vi "Fuel Injector Stage Voltage Threshold.vi"(8 "error in (no error)":errorcluster, 11 "Node Ptr":T1 format="%.0x") -> (0 "error out":errorcluster)   [LabVIEW 2019, in "Fuel Injector Analysis Addon System Explorer.lvlib"]
uses:
  Fuel Injector Analysis Addon System Explorer.lvlib
  <vilib>/NI VeriStand/Custom Device API/Custom Device Item Ref.ctl
  <vilib>/NI VeriStand/Custom Device API/Custom Device API.lvlib
panel:
  out "Units":string
  in  "Default Value":dbl
  in  "SHDocVw.IWebBrowser":refnum<k7>(container)
  in  "Header":cluster{"Section Name":string}={"Section Name"="Custom Device Item Settings"}
  in  "Description":string
  out "Name":string
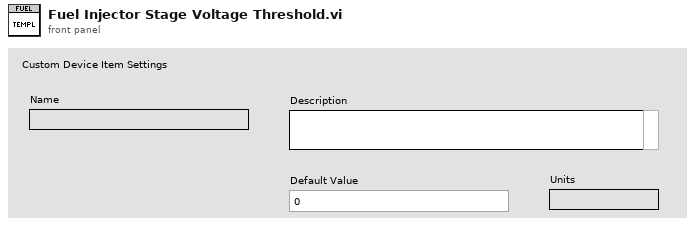
[diagram p1: front panel]
types:
  T1 = typedef "Custom Device API.lvlib/Custom Device Item Ref.ctl" = u64
  T2 = typedef "Custom Device API.lvlib/Custom Device Channel.ctl" = cluster{"Type":T3, "Units":string, "Default Value":dbl, "Faultable":bool, "Scalable":bool}
  T3 = typedef "Custom Device API.lvlib/Custom Device Channel Type.ctl" = enum16{"Input", "Output"}
  T4 = typedef "Custom Device API.lvlib/Custom Device Commands.ctl" = enum16{"Default", "Item renamed", "Shutdown", "Dynamic button pressed"}
  T5 = typedef "Custom Device API.lvlib/Custom Device Item Info.ctl" = cluster{"Name":string, "Is Channel":bool, "GUID":string, "Is Waveform":bool}
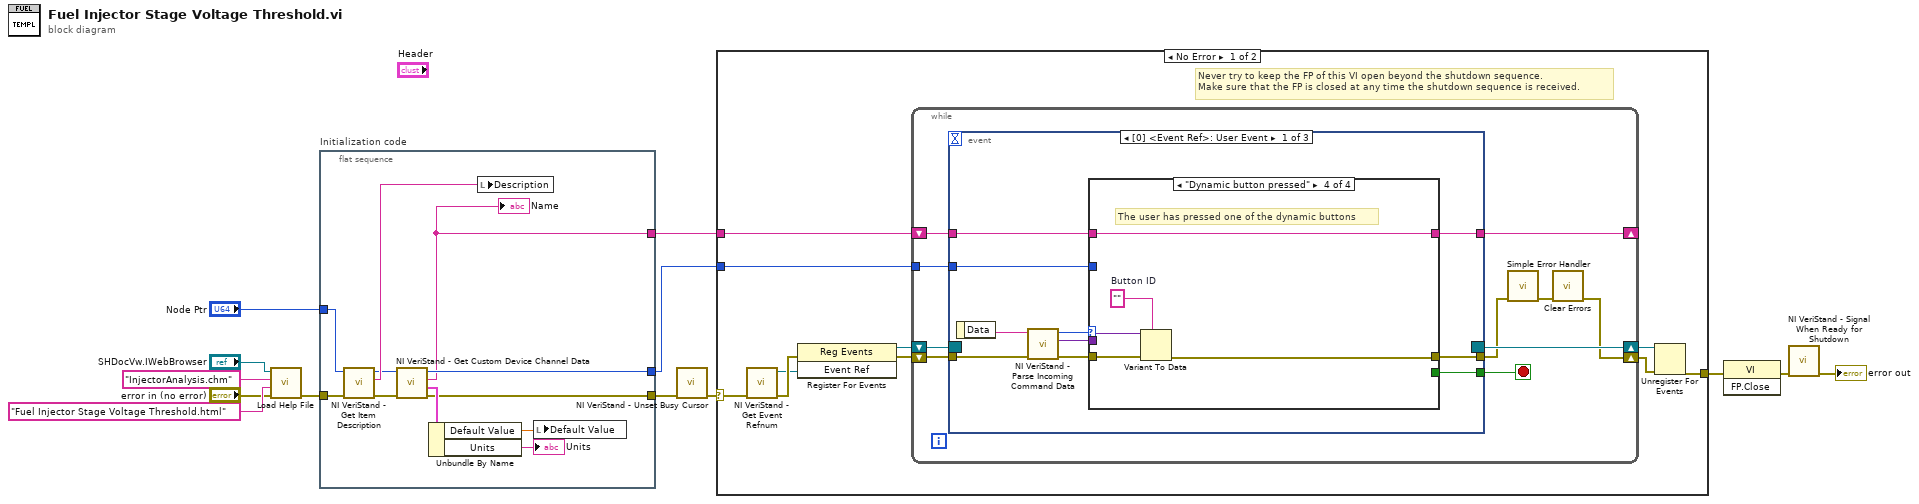
[diagram p0: block diagram]
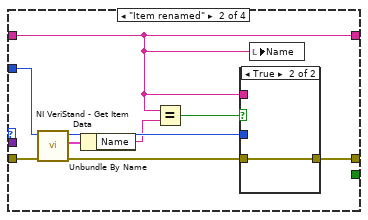
[diagram p3: hidden frame]
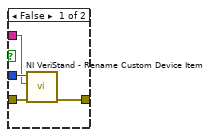
[diagram p4: hidden frame]
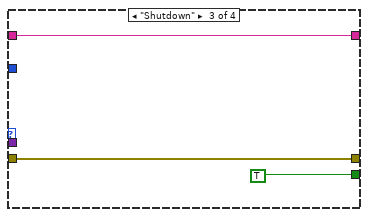
[diagram p5: hidden frame]
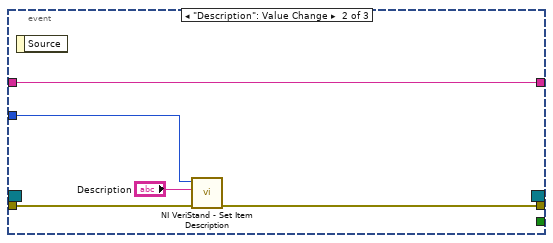
[diagram p6: hidden frame]
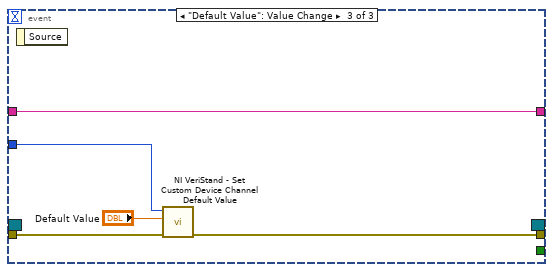
[diagram p7: hidden frame]
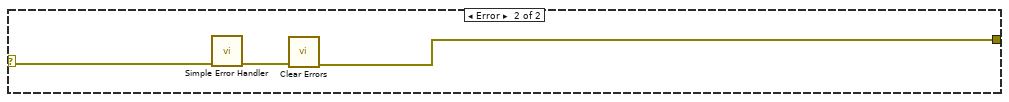
[diagram p8: hidden frame]
diagram:
  n1 = call "Load Help File.vi"("error in (no error)"="error in (no error)", "HTML File"="Fuel Injector Stage Voltage Threshold.html", "Main CHM File"="InjectorAnalysis.chm", "SHDocVw.IWebBrowser2"="SHDocVw.IWebBrowser") -> ("error out"=w4:errorcluster)  [unwired: 7 in]
  n2 = flat-sequence "Initialization code" {
    tunnel: w4 -> [w24]
    tunnel: [w14] -> w10
    tunnel: [w21] -> w8
    tunnel: "Node Ptr" -> [w22]
    tunnel: [w15] -> w1
    frame #0 {
      n3 = call <vilib>:"NI VeriStand - Get Item Description.vi"("error in (no error)"=w24, "Item Ref in"=w22) -> ("error out"=w20:errorcluster, "Description"=w23:string, "Item Ref out"=w19:T1)  [unwired: 7 out]
      n4 = call <vilib>:"NI VeriStand - Get Custom Device Channel Data.vi"("error in (no error)"=w20, "Channel Ref in"=w19) -> ("error out"=w14:errorcluster, "Channel"=w18:T2, "Channel Name"=w15:string, "Channel Ref out"=w21:T1)  [unwired: 4 in, 2 out]
      "Name" <- w15
      n5 = Unbundle By Name(w18) -> ("Default Value"=w16:dbl, "Units"=→"Units":string)
      n6 = local write "Description"(w23) -> ()
      n7 = local write "Default Value"(w16) -> ()
    }
  }
  n8 = call <vilib>:"NI VeriStand - Unset Busy Cursor.vi"("error in (no error)"=w10) -> ("error out"=w9:errorcluster)  [unwired: 10 out]
  n9 = case shown="No Error" w9 {
    selector: w9 -> [w26 w91]
    tunnel: [w31 w89] -> w13
    tunnel: w8 -> [w27 _]
    tunnel: w1 -> [w25 _]
    frame No Error {
      # "Never try to keep the FP of this VI open beyond the shutdown sequence.\nMake sure that the FP is closed at any time the shutdown sequence is received."
      n10 = call <vilib>:"NI VeriStand - Get Event Refnum.vi"("error in (no error)"=w26) -> ("error out"=w34:errorcluster, "Event Ref"=w30:refnum<user-event>)  [unwired: 9 out]
      n11 = register-events(error in=w34, w30) -> (reference out=w28:refnum<event-registration>, error out=w29:errorcluster)  [unwired: 1 in]
      n12 = while {
        tunnel: w27 -> [w40]
        shift-right: [w37] -> w32
        shift-left: w29 -> [w43]
        shift-right: [w44] -> w33
        shift-left: w28 -> [w42]
        shift-right: [w35] -> _
        shift-left: w25 -> [w36]
        stop <- w41 stop-if-true
        n13 = event shown="[0] <Event Ref>: User Event" {
          selector: w42 -> [_ _ _]
          dyn-events: [_ _ _] -> w44
          timeout: _ -> [_ _ _]
          tunnel: w43 -> [w54 w82 w88]
          tunnel: [w50 _ _] -> w41
          tunnel: [w49 w81 w87] -> w39
          tunnel: w40 -> [w48 w83 w85]
          tunnel: w36 -> [w46 w79 w84]
          tunnel: [w45 w79 w84] -> w35
          event User Event {
            n14 = event-data() -> ("Data"=w53:string)  [unwired: 1 out]
            n15 = call <vilib>:"NI VeriStand - Parse Incoming Command Data.vi"("error in (no error)"=w54, "Incoming data"=w53) -> ("error out"=w52:errorcluster, "Outgoing data"=w47:variant, "Action"=w51:T4)  [unwired: 7 out]
            n16 = case shown="\"Dynamic button pressed\"" w51 {
              tunnel: w52 -> [w56 w62 w72 w78]
              tunnel: [_ _ TRUE _] -> w50
              tunnel: [w56 w65 w72 w75] -> w49
              tunnel: w48 -> [_ w63 _ _]
              tunnel: w47 -> [_ _ _ w77]
              tunnel: w46 -> [w55 w57 w71 w74]
              tunnel: [w55 w57 w71 w74] -> w45
              frame "Default", Default {
              }
              frame "Item renamed" {
                n17 = call <vilib>:"NI VeriStand - Get Item Data.vi"("error in (no error)"=w62, "Item Ref in"=w63) -> ("error out"=w61:errorcluster, "Item Info"=w64:T5, "Item Ref out"=w60:T1)  [unwired: 7 out]
                n18 = Unbundle By Name(w64) -> ("Name"=w59:string)
                n19 = Equal?(x=w57, y=w59) -> (x = y?=w58:bool)
                n20 = case shown="True" w58 {
                  tunnel: [w69 w70] -> w65
                  tunnel: w61 -> [w68 w70]
                  tunnel: w60 -> [w67 _]
                  tunnel: w57 -> [w66 _]
                  frame False {
                    n21 = call <vilib>:"NI VeriStand - Rename Custom Device Item.vi"("error in (no error)"=w68, "New Name"=w66, "Item Ref in"=w67) -> ("error out"=w69:errorcluster)  [unwired: 6 in, 2 out]
                  }
                  frame True {
                  }
                }
                n22 = local write "Name"(w57) -> ()
              }
              frame "Shutdown" {
              }
              frame "Dynamic button pressed" {
                w76 = ""  # Button ID
                # "The user has pressed one of the dynamic buttons"
                n23 = Variant To Data(error in=w78, type=w76, Variant=w77) -> (error out=w75:errorcluster)  [unwired: 1 out]
              }
            }
          }
          event "Description": Value Change {
            n24 = event-data() -> ()  [unwired: 2 out]
            n25 = call <vilib>:"NI VeriStand - Set Item Description.vi"("error in (no error)"=w82, "Description"="Description", "Item Ref in"=w83) -> ("error out"=w81:errorcluster)  [unwired: 8 out]
          }
          event "Default Value": Value Change {
            n26 = event-data() -> ()  [unwired: 2 out]
            n27 = call <vilib>:"NI VeriStand - Set Custom Device Channel Default Value.vi"("error in (no error)"=w88, "Default Value"="Default Value", "Channel Ref in"=w85) -> ("error out"=w87:errorcluster)  [unwired: 7 in, 1 out]
          }
        }
        n28 = call <vilib>:"Simple Error Handler.vi"("error in (no error)"=w39) -> ("error out"=w38:errorcluster)  [unwired: 1 in, 7 out]
        n29 = call <vilib>:"Clear Errors.vi"("error in (no error)"=w38) -> ("error out"=w37:errorcluster)  [unwired: 1 in, 5 out]
      }
      n30 = Unregister For Events(event registration refnum=w33, error in=w32) -> (error out=w31:errorcluster)
    }
    frame Error {
      n31 = call <vilib>:"Simple Error Handler.vi"("error in (no error)"=w91) -> ("error out"=w90:errorcluster)  [unwired: 1 in, 7 out]
      n32 = call <vilib>:"Clear Errors.vi"("error in (no error)"=w90) -> ("error out"=w89:errorcluster)  [unwired: 1 in, 5 out]
    }
  }
  n33 = invoke class="VI" method="FP.Close"(error in=w13) -> (error out=w12:errorcluster)  [unwired: 2 in, 2 out]
  n34 = call <vilib>:"NI VeriStand - Signal When Ready for Shutdown.vi"("error in (no error)"=w12) -> ("error out"=→"error out":errorcluster)  [unwired: 10 out]
